vi "Update Head Position.vi"(9 "Direction":string, 10 "Update?":bool, 11 "Head Position in":T1) -> (3 "Head Position out":T1)   [LabVIEW 2021]
uses:
  Positions.ctl
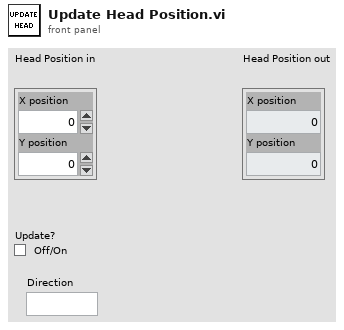
[diagram p1: front panel]
types:
  T1 = typedef "Positions.ctl" = cluster{"X position":i32, "Y position":i32}
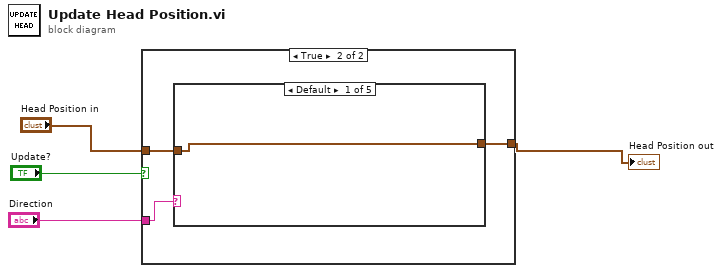
[diagram p0: block diagram]
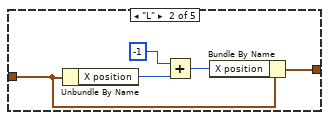
[diagram p3: hidden frame]
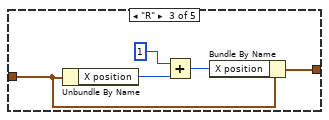
[diagram p4: hidden frame]
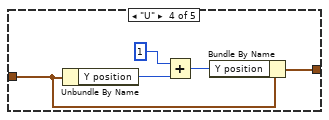
[diagram p5: hidden frame]
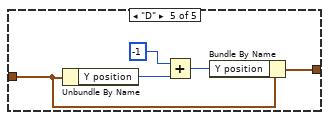
[diagram p6: hidden frame]
diagram:
  n1 = case shown="True" "Update?" {
    tunnel: "Head Position in" -> [w5 w8]
    tunnel: [w5 w7] -> w3
    tunnel: "Direction" -> [_ w6]
    frame False {
    }
    frame True {
      n2 = case shown="Default" w6 {
        tunnel: w8 -> [w9 w11 w16 w21 w26]
        tunnel: [w9 w10 w15 w20 w25] -> w7
        frame Default {
        }
        frame "L" {
          n3 = Unbundle By Name(w11) -> ("X position"=w14:i32)
          n4 = Add(x=-1, y=w14) -> (x+y=w13:i32)
          n5 = Bundle By Name(cluster=w11, "X position"=w13) -> (w10:T1)
        }
        frame "R" {
          n6 = Unbundle By Name(w16) -> ("X position"=w19:i32)
          n7 = Add(x=1, y=w19) -> (x+y=w18:i32)
          n8 = Bundle By Name(cluster=w16, "X position"=w18) -> (w15:T1)
        }
        frame "U" {
          n9 = Unbundle By Name(w21) -> ("Y position"=w24:i32)
          n10 = Add(x=1, y=w24) -> (x+y=w23:i32)
          n11 = Bundle By Name(cluster=w21, "Y position"=w23) -> (w20:T1)
        }
        frame "D" {
          n12 = Unbundle By Name(w26) -> ("Y position"=w29:i32)
          n13 = Add(x=-1, y=w29) -> (x+y=w28:i32)
          n14 = Bundle By Name(cluster=w26, "Y position"=w28) -> (w25:T1)
        }
      }
    }
  }
  "Head Position out" <- w3
